vi "GetNewLogFilePath.vi"(8 "error in (no error)":errorcluster) -> (0 "error out":errorcluster, 2 "New log filename":string, 3 "New log file path":path)   [LabVIEW 2013]
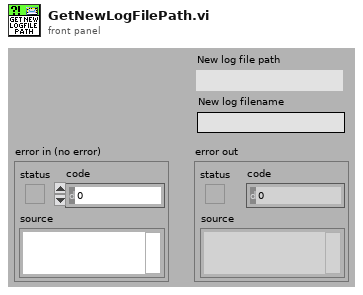
[diagram p1: front panel]
types:
  T1 = typedef "ApplicationPaths.ctl" = cluster{"Data Path":path, "Log Path":path, "Tmp Path":path}
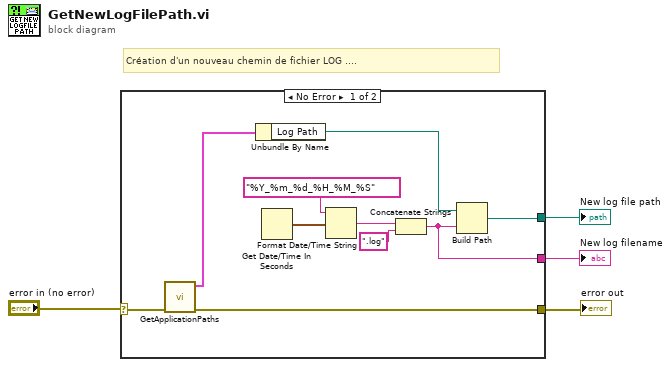
[diagram p0: block diagram]
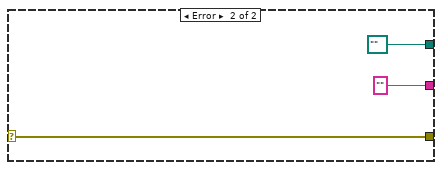
[diagram p2: hidden frame]
diagram:
  # "Création d'un nouveau chemin de fichier LOG ...."
  n1 = case shown="No Error" "error in (no error)" {
    selector: "error in (no error)" -> [w14 w17]
    tunnel: [w6 w17] -> w3
    tunnel: [w7 path "" ("New log file path")] -> w2
    tunnel: [w5 ""] -> w1
    frame No Error {
      n2 = call "GetApplicationPaths.vi"("error in (no error)"=w14) -> ("error out"=w6:errorcluster, "ApplicationPath"=w13:T1)  [unwired: 9 in]
      n3 = Unbundle By Name(w13) -> ("Log Path"=w8:path)
      n4 = Get Date/Time In Seconds() -> (seconds since 1Jan1904=w12:timestamp)
      n5 = Format Date/Time String(time format string (%c)="%Y_%m_%d_%H_%M_%S", seconds (now)=w12) -> (date/time string=w10:string)  [unwired: 1 in]
      n6 = Concatenate Strings(w10, ".log" ("string")) -> (w5:string)
      n7 = Build Path(base path=w8, name or relative path=w5) -> (appended path=w7:path)
    }
    frame Error {
    }
  }
  "error out" <- w3
  "New log file path" <- w2
  "New log filename" <- w1
